vi "CLSUIP_Read Future Parent ProjectItem.vi"(8 "error in (no error)":errorcluster, 11 "VIRetooler in":refnum<class "VIRetooler.lvclass">) -> (0 "error out":errorcluster, 2 "Future Parent ProjectItem":refnum<vi>, 3 "VIRetooler out":refnum<class "VIRetooler.lvclass">)   [LabVIEW 2021, in "MemberVICreation.lvlib" / "VIRetooler.lvclass"]
uses:
  <resource>/Framework/Providers/LVClassLibrary/NewAccessors/VIRetooler/VIRetooler.lvclass
  <resource>/Framework/Providers/LVClassLibrary/NewAccessors/VIRetooler/VIRetooler.lvclass/VIRetooler.ctl
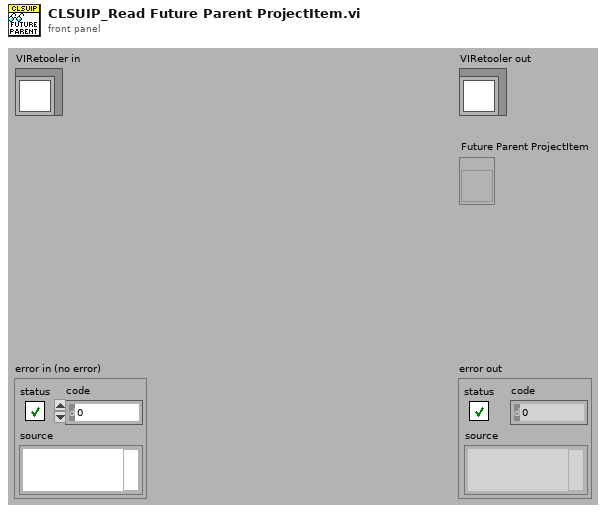
[diagram p1: front panel]
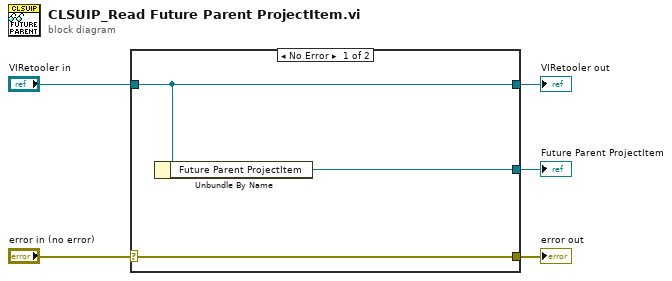
[diagram p0: block diagram]
diagram:
  n1 = case shown="No Error" "error in (no error)" {
    selector: "error in (no error)" -> [w8 w9]
    tunnel: [w8 w9] -> w4
    tunnel: [w7 w10] -> w2
    tunnel: "VIRetooler in" -> [w7 w10]
    tunnel: [w6 _] -> w1
    frame No Error {
      n2 = Unbundle By Name(w7) -> ("Future Parent ProjectItem"=w6:refnum<vi>)
    }
    frame Error {
    }
  }
  "error out" <- w4
  "VIRetooler out" <- w2
  "Future Parent ProjectItem" <- w1
